vi "reconstructObject.vi"(9 "ctrlFactor":dbl, 10 "objRef":dbl[][](graph), 11 "imgRaw":dbl[][](graph)) -> (0 "error out":errorcluster, 1 "Frame count":dbl, 2 "objPro":dbl[][](graph), 3 "imgPro":dbl[][](graph))   [LabVIEW 2016]
uses:
  <vilib>/Utility/error.llb/DialogType.ctl
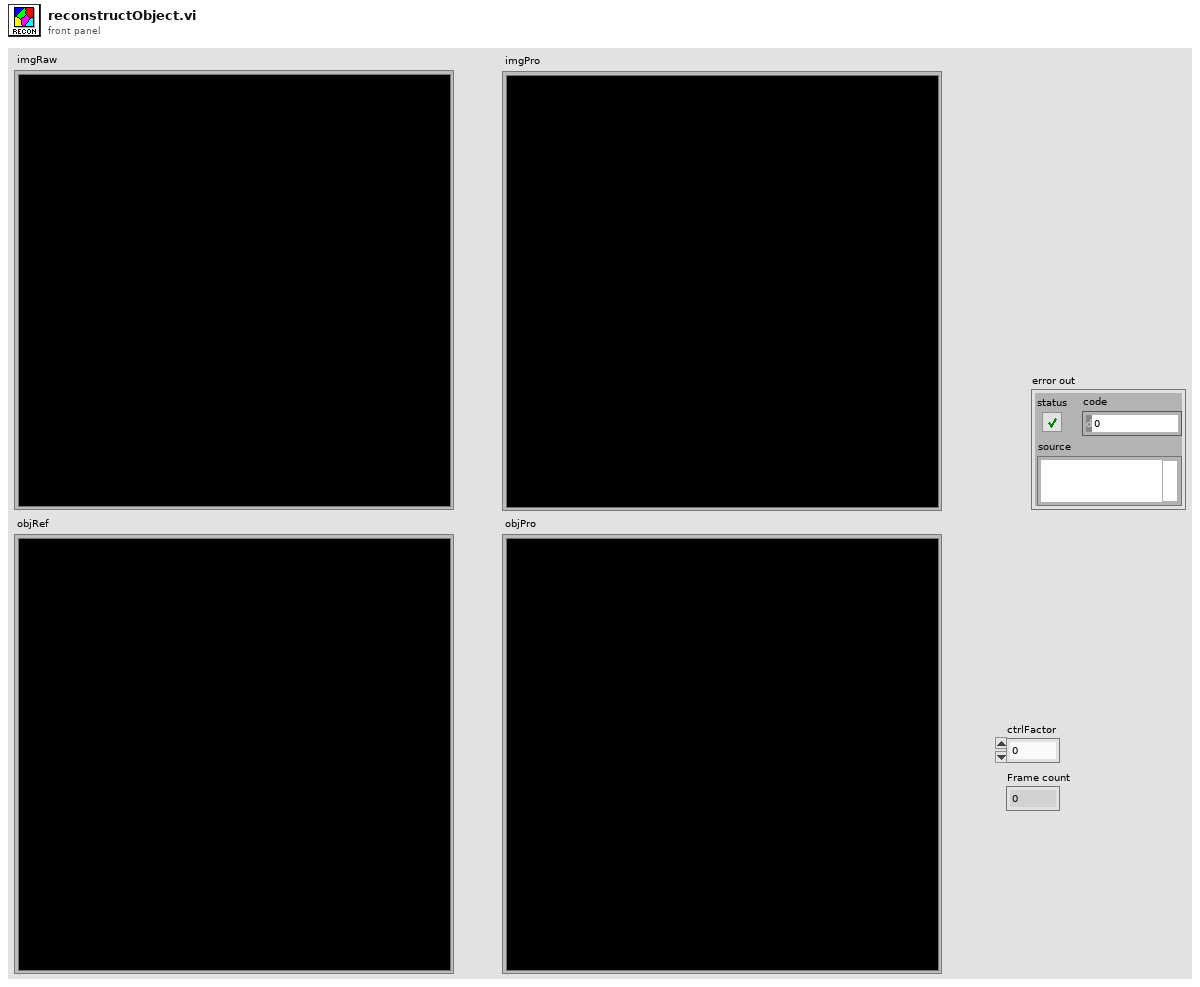
[diagram p1: front panel]
types:
  T1 = typedef "DialogType.ctl" = u16
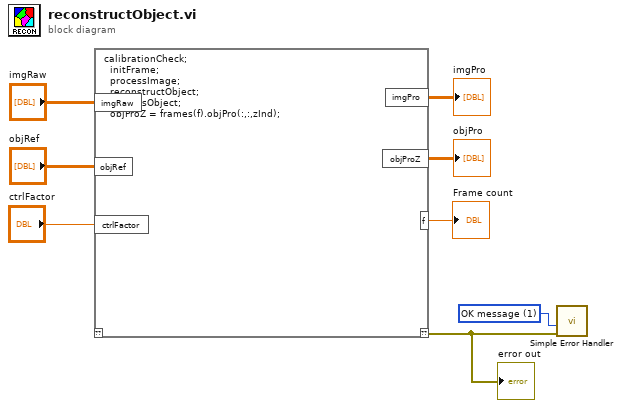
[diagram p0: block diagram]
diagram:
  w1 = T1 1 items=["no dialog", "OK message", "continue or stop message", "OK message + warnings", "continue/stop + warnings"] ("type of dialog (OK msg:1)")
  n1 = script code="calibrationCheck;\n  initFrame;\n  processImage;\n  reconstructObject;\n  processObject;\n  objProZ = frames(f).objPro(:,:,zInd);"("imgRaw"="imgRaw", "objRef"="objRef", "ctrlFactor"="ctrlFactor") -> ("??"=w2:errorcluster, "imgPro"=→"imgPro":dbl[][], "objProZ"=→"objPro":dbl[][], "f"=→"Frame count":dbl)  [unwired: 1 in]
  "error out" <- w2
  n2 = call <vilib>:"Simple Error Handler.vi"("type of dialog (OK msg:1)"=w1, "error in (no error)"=w2) -> ()  [unwired: 3 in, 5 out]
